vi "1108_JoystickPantherDriveMapping.vi"(9 "x-spin":dbl min=-1.0 max=1.0 step=0.1, 10 "y":dbl min=-1.0 max=1.0 step=0.1, 11 "x":dbl min=-1.0 max=1.0 step=0.1) -> (0 "Motor RR":dbl, 1 "Motor FR":dbl, 2 "Motor FL":dbl, 3 "Motor RL":dbl, 4 "theta":dbl=90.0)   [LabVIEW 2018]
doc: "Maps the joystick inputs for holonomic driving. Holonomic driving allows you to move the robot in any direction without first rotating or maneuvering the robot.\n\nThis VI assumes the robot to have either four omni-directional wheels and four motors mounted at 45 degree angles in the four corners of a square frame or to have four mecanum wheels driven by four motors."
uses:
  <vilib>/Analysis/coordinate.llb/Angle Units.ctl
  <vilib>/Analysis/coordinate.llb/Angle Range (Degree).ctl
  <vilib>/Analysis/coordinate.llb/Angle Rotation (scalar).vi
  <vilib>/Analysis/coordinate.llb/Wrap Angle (scalar).vi
  <vilib>/Analysis/NI_AAL_Angle.lvlib
panel:
  out "theta_out":dbl
  in  "180 drive?":bool=TRUE
  out "power":dbl
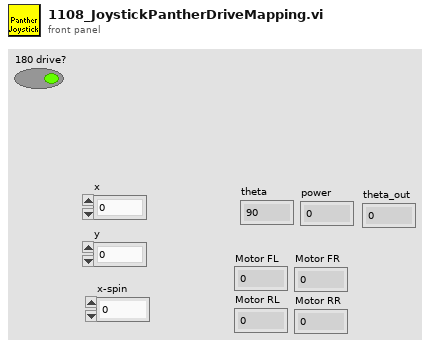
[diagram p1: front panel]
types:
  T1 = typedef "NI_AAL_Angle.lvlib/Angle Range (Degree).ctl" = u16
  T2 = typedef "NI_AAL_Angle.lvlib/Angle Units.ctl" = i32
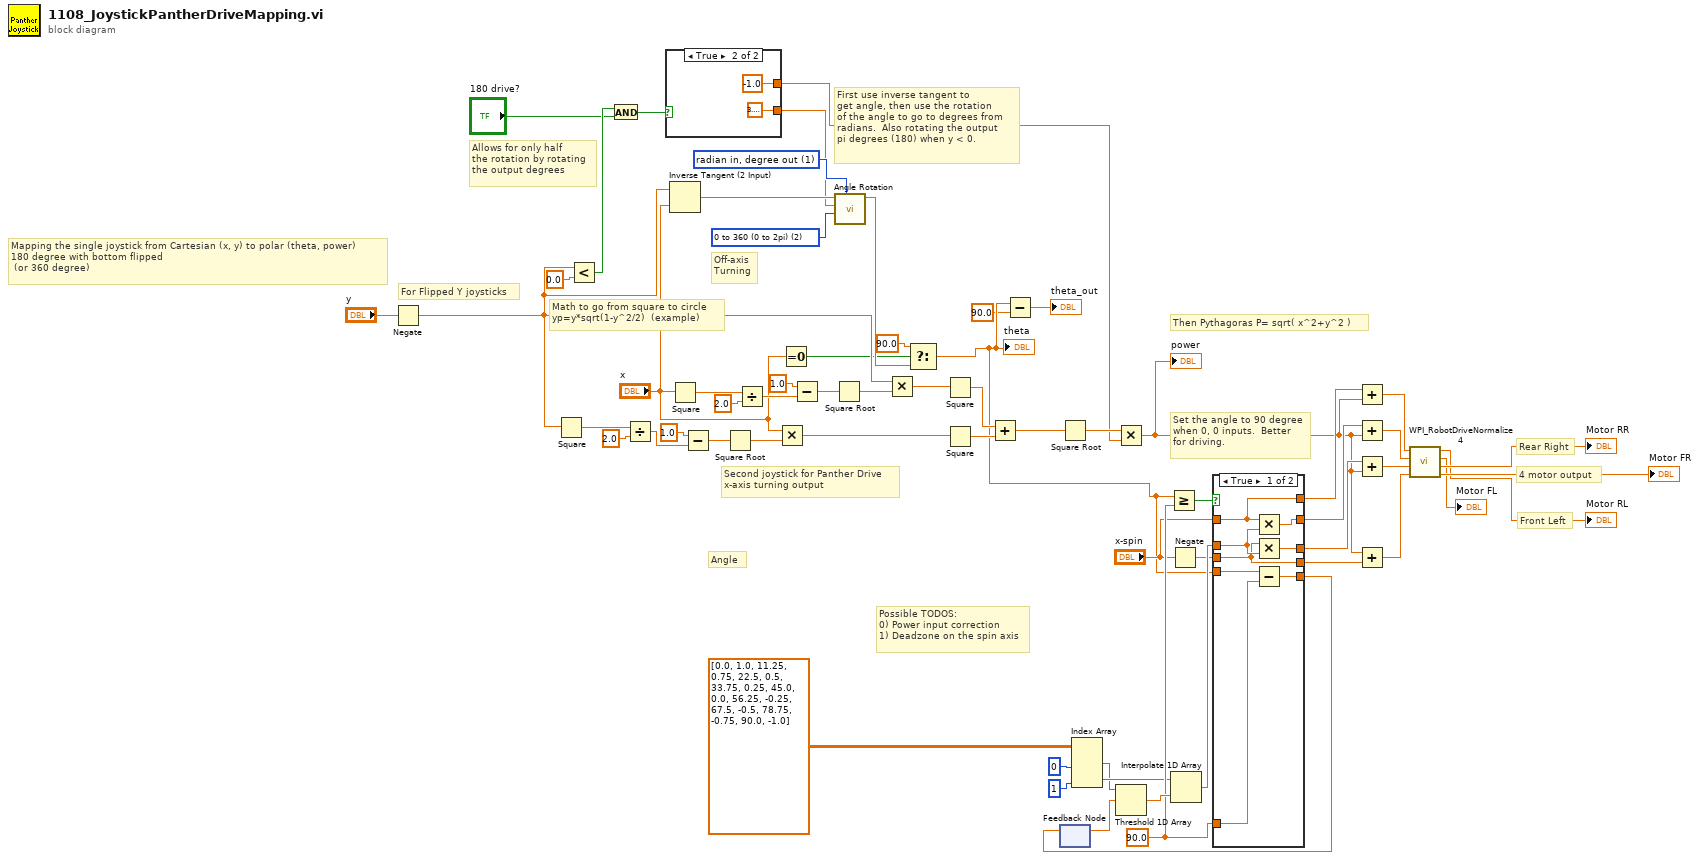
[diagram p0: block diagram]
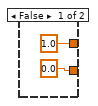
[diagram p2: hidden frame]
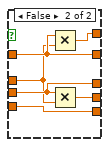
[diagram p3: hidden frame]
diagram:
  w35 = T1 2 items=["none", "-180 to 180 (-pi to pi)", "0 to 360 (0 to 2pi)"] ("rotated angle range")
  w37 = T2 1 items=["radian in, radian out", "radian in, degree out", "degree in, degree out", "degree in, radian out"] ("angle units")
  w60 = 90.0 ("y")
  # "Mapping the single joystick from Cartesian (x, y) to polar (theta, power)\n180 degree with bottom flipped\n (or 360 degree)"
  # "Set the angle to 90 degree\nwhen 0, 0 inputs.  Better\nfor driving."
  # "First use inverse tangent to \nget angle, then use the rotation\nof the angle to go to degrees from\nradians.  Also rotating the output\npi degrees (180) when y < 0."
  # "Then Pythagoras P= sqrt( x^2+y^2 )"
  # "Math to go from square to circle\nyp=y*sqrt(1-y^2/2)  (example)"
  # "Allows for only half\nthe rotation by rotating\nthe output degrees"
  # "For Flipped Y joysticks"
  # "Front Left"
  # "Rear Right"
  # "4 motor output"
  # "Off-axis\nTurning"
  # "Possible TODOS:  \n0) Power input correction\n1) Deadzone on the spin axis"
  # "Angle"
  # "Second joystick for Panther Drive\nx-axis turning output"
  n1 = Negate(x="y") -> (-x=w17:dbl)
  n2 = Square(x=w17) -> (x^2=w31:dbl)
  n3 = Less?(x=w17, y=0.0) -> (x < y?=w13:bool)
  n4 = And(x=w13, y="180 drive?") -> (x .and. y?=w14:bool)
  n5 = Divide(x=w31, y=2.0) -> (x/y=w20:dbl)
  n6 = case shown="True" w14 {
    tunnel: [0.0 ("counterclockwise rotation") 3.141592653589793] -> w16
    tunnel: [1.0 -1.0] -> w5
    frame False {
    }
    frame True {
    }
  }
  n7 = Inverse Tangent (2 Input)(1:"x", 2:w17) -> (0:w36:dbl)
  n8 = Square(x="x") -> (x^2=w26:dbl)
  n9 = Subtract(x=1.0, y=w20) -> (x-y=w29:dbl)
  n10 = Square Root(x=w29) -> (sqrt(x)=w28:dbl)
  n11 = Divide(x=w26, y=2.0) -> (x/y=w27:dbl)
  n12 = Multiply(x="x", y=w28) -> (x*y=w18:dbl)
  n13 = Equal To 0?(x="x") -> (x = 0?=w7:bool)
  n14 = Subtract(x=1.0, y=w27) -> (x-y=w24:dbl)
  n15 = Square Root(x=w24) -> (sqrt(x)=w22:dbl)
  n16 = call-poly <vilib>:"Angle Rotation.vi"("angle units"=w37, "rotated angle range"=w35, "counterclockwise rotation"=w16, "angle"=w36) -> ("rotated angle"=w8:dbl)  [unwired: 6 in, 1 out]
  n17 = Multiply(x=w17, y=w22) -> (x*y=w19:dbl)
  n18 = Select(t=90.0, s=w7, f=w8) -> (s? t:f=w3:dbl)
  "theta" <- w3
  n19 = Square(x=w19) -> (x^2=w33:dbl)
  n20 = Square(x=w18) -> (x^2=w34:dbl)
  n21 = Add(x=w33, y=w34) -> (x+y=w32:dbl)
  n22 = Subtract(x=w3, y=90.0) -> (x-y=→"theta_out":dbl)
  n23 = Square Root(x=w32) -> (sqrt(x)=w6:dbl)
  n24 = feedback #1() -> (w58:dbl)  [unwired: 1 in]
  n25 = Index Array(array=sgl[][] [[0.0, 1.0], [11.25, 0.75], [22.5, 0.5], [33.75, 0.25], [45.0, 0.0], [56.25, -0.25], [67.5, -0.5], [78.75, -0.75], [90.0, -1.0]], index (col) #1=0 ("disabled index (col)"), index (col) #2=1 ("index (col)")) -> (element #1=w50:sgl[], element #2=w51:sgl[])  [unwired: 2 in]
  n26 = Multiply(x=w6, y=w5) -> (x*y=w4:dbl)
  "power" <- w4
  n27 = Threshold 1D Array(2:w58, 3:w50) -> (0:w62:sgl)  [unwired: 1 in]
  n28 = Greater Or Equal?(x=w3, y=w60) -> (x >= y?=w61:bool)
  n29 = Negate(x="x-spin") -> (-x=w55:dbl)
  n30 = Interpolate 1D Array(1:w62, 2:w51) -> (0:w59:sgl)
  n31 = case shown="True" w61 {
    tunnel: w3 -> [w74 w78]
    tunnel: [w73 w78] -> w57
    tunnel: w60 -> [w72 _]
    tunnel: w59 -> [w69 w75]
    tunnel: [w71 w80] -> w44
    tunnel: [w67 w76] -> w42
    tunnel: [w70 w77] -> w45
    tunnel: [w68 w79] -> w43
    tunnel: w55 -> [w67 w79]
    tunnel: "x-spin" -> [w70 w80]
    frame True {
      n32 = Multiply(x=w70, y=w69) -> (x*y=w71:dbl)
      n33 = Multiply(x=w67, y=w69) -> (x*y=w68:dbl)
      n34 = Subtract(x=w74, y=w72) -> (x-y=w73:dbl)
    }
    frame False {
      n35 = Multiply(x=w80, y=w75) -> (x*y=w77:dbl)
      n36 = Multiply(x=w79, y=w75) -> (x*y=w76:dbl)
    }
  }
  n37 = feedback-in #1(w57) -> ()
  n38 = Add(x=w45, y=w4) -> (x+y=w46:dbl)
  n39 = Add(x=w44, y=w4) -> (x+y=w47:dbl)
  n40 = Add(x=w43, y=w4) -> (x+y=w48:dbl)
  n41 = Add(x=w4, y=w42) -> (x+y=w49:dbl)
  n42 = call <vilib>:"WPI_RobotDriveNormalize 4.vi"("D"=w49, "C"=w48, "B"=w47, "A"=w46) -> ("D'"=→"Motor FR":dbl, "C'"=→"Motor RR":dbl, "B'"=→"Motor FL":dbl, "A'"=→"Motor RL":dbl)
